vi "CAN_LIN_FlexRay_Demo_Template.vi"() -> ()   [LabVIEW 2014]
uses:
  TSMaster_API/LIN_Function/Typedef/TSLIN_Transmit.ctl
  TSMaster_API/CAN_CANFD_Function/Typedef/TLibCANFD.ctl
  TSMaster_API/LIN_Function/Typedef/TLibLIN.ctl
  TSMaster_API/FlexRay_Function/Typedef/TLibFLexRay.ctl
panel:
  out "FR_Buffer":T1[](array[typedef])
  out "ACANMsgBuffer":T2(array[cluster])
  out "ALINBuffer":T3[](array[typedef])
  # "使用方法：\n1.创建TSMaster 工程，映射CAN/LIN/FlexRay通道2，并开启接收Trace\n2.此demo 映射通道1\n3.通道1与通道2进行短接\n4.运行此demo 发送Fdata ,并接收Fdata"
  # "usage method:\n1. Create TSMaster project, map CAN/LIN/FlexRay channel 2, and enable receiving Trace. \n2. This demo maps channel 1. \n3. Short circuit channel 1 to channel 2\n4. Run this demo sends and receives Fdata"
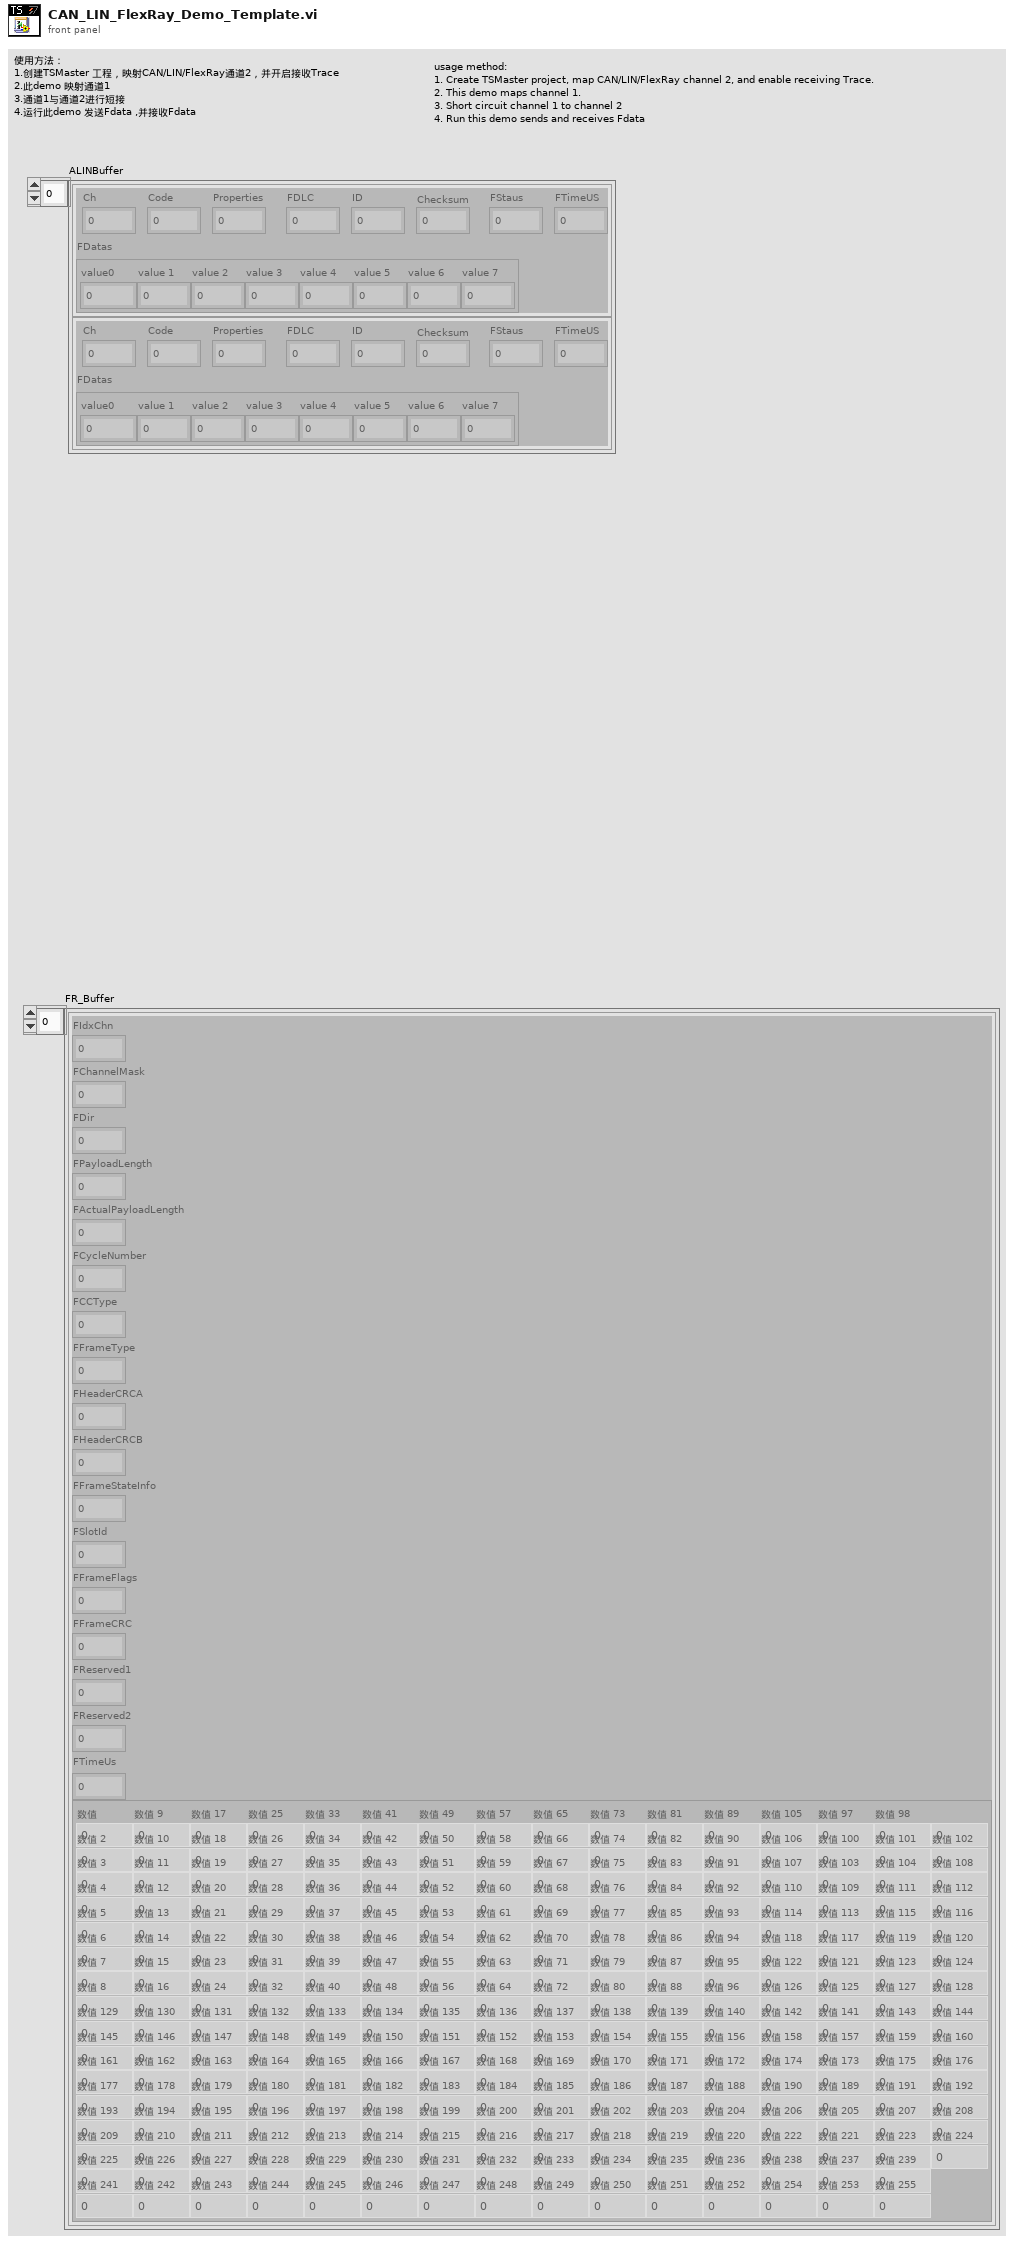
[diagram p1: front panel]
types:
  T1 = typedef "TLibFLexRay.ctl" = cluster{"FIdxChn":u8, "FChannelMask":u8, "FDir":u8, "FPayloadLength":u8, "FActualPayloadLength":u8, "FCycleNumber":u8, "FCCType":u8, "FFrameType":u8, "FHeaderCRCA":u16, "FHeaderCRCB":u16, "FFrameStateInfo":u16, "FSlotId":u16, "FFrameFlags":u32, "FFrameCRC":u32, "FReserved1":u64, "FReserved2":u64, "FTimeUs":u64, "FData":cluster{"数值":u8, "数值 9":u8, "数值 17":u8, "数值 25":u8, "数值 33":u8, "数值 41":u8, "数值 49":u8, "数值 57":u8, "数值 65":u8, "数值 73":u8, "数值 81":u8, "数值 89":u8, "数值 97":u8, "数值 105":u8, "数值 98":u8, "数值 99":u8, "数值 2":u8, "数值 10":u8, "数值 18":u8, "数值 26":u8, "数值 34":u8, "数值 42":u8, "数值 50":u8, "数值 58":u8, "数值 66":u8, "数值 74":u8, "数值 82":u8, "数值 90":u8, "数值 100":u8, "数值 106":u8, "数值 101":u8, "数值 102":u8, "数值 3":u8, "数值 11":u8, "数值 19":u8, "数值 27":u8, "数值 35":u8, "数值 43":u8, "数值 51":u8, "数值 59":u8, "数值 67":u8, "数值 75":u8, "数值 83":u8, "数值 91":u8, "数值 103":u8, "数值 107":u8, "数值 104":u8, "数值 108":u8, "数值 4":u8, "数值 12":u8, "数值 20":u8, "数值 28":u8, "数值 36":u8, "数值 44":u8, "数值 52":u8, "数值 60":u8, "数值 68":u8, "数值 76":u8, "数值 84":u8, "数值 92":u8, "数值 109":u8, "数值 110":u8, "数值 111":u8, "数值 112":u8, "数值 5":u8, "数值 13":u8, "数值 21":u8, "数值 29":u8, "数值 37":u8, "数值 45":u8, "数值 53":u8, "数值 61":u8, "数值 69":u8, "数值 77":u8, "数值 85":u8, "数值 93":u8, "数值 113":u8, "数值 114":u8, "数值 115":u8, "数值 116":u8, "数值 6":u8, "数值 14":u8, "数值 22":u8, "数值 30":u8, "数值 38":u8, "数值 46":u8, "数值 54":u8, "数值 62":u8, "数值 70":u8, "数值 78":u8, "数值 86":u8, "数值 94":u8, "数值 117":u8, "数值 118":u8, "数值 119":u8, "数值 120":u8, "数值 7":u8, "数值 15":u8, "数值 23":u8, "数值 31":u8, "数值 39":u8, "数值 47":u8, "数值 55":u8, "数值 63":u8, "数值 71":u8, "数值 79":u8, "数值 87":u8, "数值 95":u8, "数值 121":u8, "数值 122":u8, "数值 123":u8, "数值 124":u8, "数值 8":u8, "数值 16":u8, "数值 24":u8, "数值 32":u8, "数值 40":u8, "数值 48":u8, "数值 56":u8, "数值 64":u8, "数值 72":u8, "数值 80":u8, "数值 88":u8, "数值 96":u8, "数值 125":u8, "数值 126":u8, "数值 127":u8, "数值 128":u8, "数值 129":u8, "数值 130":u8, "数值 131":u8, "数值 132":u8, "数值 133":u8, "数值 134":u8, "数值 135":u8, "数值 136":u8, "数值 137":u8, "数值 138":u8, "数值 139":u8, "数值 140":u8, "数值 141":u8, "数值 142":u8, "数值 143":u8, "数值 144":u8, "数值 145":u8, "数值 146":u8, "数值 147":u8, "数值 148":u8, "数值 149":u8, "数值 150":u8, "数值 151":u8, "数值 152":u8, "数值 153":u8, "数值 154":u8, "数值 155":u8, "数值 156":u8, "数值 157":u8, "数值 158":u8, "数值 159":u8, "数值 160":u8, "数值 161":u8, "数值 162":u8, "数值 163":u8, "数值 164":u8, "数值 165":u8, "数值 166":u8, "数值 167":u8, "数值 168":u8, "数值 169":u8, "数值 170":u8, "数值 171":u8, "数值 172":u8, "数值 173":u8, "数值 174":u8, "数值 175":u8, "数值 176":u8, "数值 177":u8, "数值 178":u8, "数值 179":u8, "数值 180":u8, "数值 181":u8, "数值 182":u8, "数值 183":u8, "数值 184":u8, "数值 185":u8, "数值 186":u8, "数值 187":u8, "数值 188":u8, "数值 189":u8, "数值 190":u8, "数值 191":u8, "数值 192":u8, "数值 193":u8, "数值 194":u8, "数值 195":u8, "数值 196":u8, "数值 197":u8, "数值 198":u8, "数值 199":u8, "数值 200":u8, "数值 201":u8, "数值 202":u8, "数值 203":u8, "数值 204":u8, "数值 205":u8, "数值 206":u8, "数值 207":u8, "数值 208":u8, "数值 209":u8, "数值 210":u8, "数值 211":u8, "数值 212":u8, "数值 213":u8, "数值 214":u8, "数值 215":u8, "数值 216":u8, "数值 217":u8, "数值 218":u8, "数值 219":u8, "数值 220":u8, "数值 221":u8, "数值 222":u8, "数值 223":u8, "数值 224":u8, "数值 225":u8, "数值 226":u8, "数值 227":u8, "数值 228":u8, "数值 229":u8, "数值 230":u8, "数值 231":u8, "数值 232":u8, "数值 233":u8, "数值 234":u8, "数值 235":u8, "数值 236":u8, "数值 237":u8, "数值 238":u8, "数值 239":u8, "数值 241":u8, "数值 242":u8, "数值 243":u8, "数值 244":u8, "数值 245":u8, "数值 246":u8, "数值 247":u8, "数值 248":u8, "数值 249":u8, "数值 250":u8, "数值 251":u8, "数值 252":u8, "数值 253":u8, "数值 254":u8, "数值 255":u8}}
  T2 = cluster{"FIdxChn":u8, "FProperties":u8, "FDLC":u8, "FReserved":u8, "FIdentifier":i32, "FTimeUS":u64, "Fdata":cluster{"初始化的数组[0]":u8, "初始化的数组[1]":u8, "初始化的数组[2]":u8, "初始化的数组[3]":u8, "初始化的数组[4]":u8, "初始化的数组[5]":u8, "初始化的数组[6]":u8, "初始化的数组[7]":u8, "初始化的数组[8]":u8, "初始化的数组[9]":u8, "初始化的数组[10]":u8, "初始化的数组[11]":u8, "初始化的数组[12]":u8, "初始化的数组[13]":u8, "初始化的数组[14]":u8, "初始化的数组[15]":u8, "初始化的数组[16]":u8, "初始化的数组[17]":u8, "初始化的数组[18]":u8, "初始化的数组[19]":u8, "初始化的数组[20]":u8, "初始化的数组[21]":u8, "初始化的数组[22]":u8, "初始化的数组[23]":u8, "初始化的数组[24]":u8, "初始化的数组[25]":u8, "初始化的数组[26]":u8, "初始化的数组[27]":u8, "初始化的数组[28]":u8, "初始化的数组[29]":u8, "初始化的数组[30]":u8, "初始化的数组[31]":u8, "初始化的数组[32]":u8, "初始化的数组[33]":u8, "初始化的数组[34]":u8, "初始化的数组[35]":u8, "初始化的数组[36]":u8, "初始化的数组[37]":u8, "初始化的数组[38]":u8, "初始化的数组[39]":u8, "初始化的数组[40]":u8, "初始化的数组[41]":u8, "初始化的数组[42]":u8, "初始化的数组[43]":u8, "初始化的数组[44]":u8, "初始化的数组[45]":u8, "初始化的数组[46]":u8, "初始化的数组[47]":u8, "初始化的数组[48]":u8, "初始化的数组[49]":u8, "初始化的数组[50]":u8, "初始化的数组[51]":u8, "初始化的数组[52]":u8, "初始化的数组[53]":u8, "初始化的数组[54]":u8, "初始化的数组[55]":u8, "初始化的数组[56]":u8, "初始化的数组[57]":u8, "初始化的数组[58]":u8, "初始化的数组[59]":u8, "初始化的数组[60]":u8, "初始化的数组[61]":u8, "初始化的数组[62]":u8, "初始化的数组[63]":u8}}[]
  T3 = typedef "TLibLIN.ctl" = cluster{"Ch":u8, "Code":u8, "Properties":u8, "FDLC":u8, "ID":u8, "Checksum":u8, "FStaus":u8, "FTimeUS":u64, "FDatas":cluster{"value0":u8, "value 1":u8, "value 2":u8, "value 3":u8, "value 4":u8, "value 5":u8, "value 6":u8, "value 7":u8}}
  T4 = cluster{"FIdxChn":u8, "FChannelMask":u8, "FActualPayloadLength":u8, "FCycleNumber":u8, "FSlotId":u16, "Send_Array":u8[]}
  T5 = enum16{"Only read received messages", "Receive&send messages"}
  T6 = typedef "TLibCANFD.ctl" = cluster{"AIdxchn":u8, "AId":i32, "AIsStd":u8, "BRS":enum16{"Close", "Open"}, "AIsData":u8, "ADLC":i32, "AIsFD":enum16{"Classic CAN Message", "FD CAN Message"}, "FDatas":cluster{"Initialize array[0]":u8, "Initialize array[1]":u8, "Initialize array[2]":u8, "Initialize array[3]":u8, "Initialize array[4]":u8, "Initialize array[5]":u8, "Initialize array[6]":u8, "Initialize array[7]":u8, "Initialize array[8]":u8, "Initialize array[9]":u8, "Initialize array[10]":u8, "Initialize array[11]":u8, "Initialize array[12]":u8, "Initialize array[13]":u8, "Initialize array[14]":u8, "Initialize array[15]":u8, "Initialize array[16]":u8, "Initialize array[17]":u8, "Initialize array[18]":u8, "Initialize array[19]":u8, "Initialize array[20]":u8, "Initialize array[21]":u8, "Initialize array[22]":u8, "Initialize array[23]":u8, "Initialize array[24]":u8, "Initialize array[25]":u8, "Initialize array[26]":u8, "Initialize array[27]":u8, "Initialize array[28]":u8, "Initialize array[29]":u8, "Initialize array[30]":u8, "Initialize array[31]":u8, "Initialize array[32]":u8, "Initialize array[33]":u8, "Initialize array[34]":u8, "Initialize array[35]":u8, "Initialize array[36]":u8, "Initialize array[37]":u8, "Initialize array[38]":u8, "Initialize array[39]":u8, "Initialize array[40]":u8, "Initialize array[41]":u8, "Initialize array[42]":u8, "Initialize array[43]":u8, "Initialize array[44]":u8, "Initialize array[45]":u8, "Initialize array[46]":u8, "Initialize array[47]":u8, "Initialize array[48]":u8, "Initialize array[49]":u8, "Initialize array[50]":u8, "Initialize array[51]":u8, "Initialize array[52]":u8, "Initialize array[53]":u8, "Initialize array[54]":u8, "Initialize array[55]":u8, "Initialize array[56]":u8, "Initialize array[57]":u8, "Initialize array[58]":u8, "Initialize array[59]":u8, "Initialize array[60]":u8, "Initialize array[61]":u8, "Initialize array[62]":u8, "Initialize array[63]":u8}}
  T7 = typedef "TSLIN_Transmit.ctl" = cluster{"Channel":i32, "Rx/TX":enum16{"Rx", "Tx"}, "Set_node_funtiontype":i32, "DLC":u32, "ID":u32, "FDatas":cluster{"value0":u8, "value 1":u8, "value 2":u8, "value 3":u8, "value 4":u8, "value 5":u8, "value 6":u8, "value 7":u8}}
  T8 = cluster{"数组[0]":u8, "数组[1]":u8, "数组[2]":u8, "数组[3]":u8, "数组[4]":u8, "数组[5]":u8, "数组[6]":u8, "数组[7]":u8, "数组[8]":u8, "数组[9]":u8, "数组[10]":u8, "数组[11]":u8, "数组[12]":u8, "数组[13]":u8, "数组[14]":u8, "数组[15]":u8, "数组[16]":u8, "数组[17]":u8, "数组[18]":u8, "数组[19]":u8, "数组[20]":u8, "数组[21]":u8, "数组[22]":u8, "数组[23]":u8, "数组[24]":u8, "数组[25]":u8, "数组[26]":u8, "数组[27]":u8, "数组[28]":u8, "数组[29]":u8, "数组[30]":u8, "数组[31]":u8, "数组[32]":u8, "数组[33]":u8, "数组[34]":u8, "数组[35]":u8, "数组[36]":u8, "数组[37]":u8, "数组[38]":u8, "数组[39]":u8, "数组[40]":u8, "数组[41]":u8, "数组[42]":u8, "数组[43]":u8, "数组[44]":u8, "数组[45]":u8, "数组[46]":u8, "数组[47]":u8, "数组[48]":u8, "数组[49]":u8, "数组[50]":u8, "数组[51]":u8, "数组[52]":u8, "数组[53]":u8, "数组[54]":u8, "数组[55]":u8, "数组[56]":u8, "数组[57]":u8, "数组[58]":u8, "数组[59]":u8, "数组[60]":u8, "数组[61]":u8, "数组[62]":u8, "数组[63]":u8}
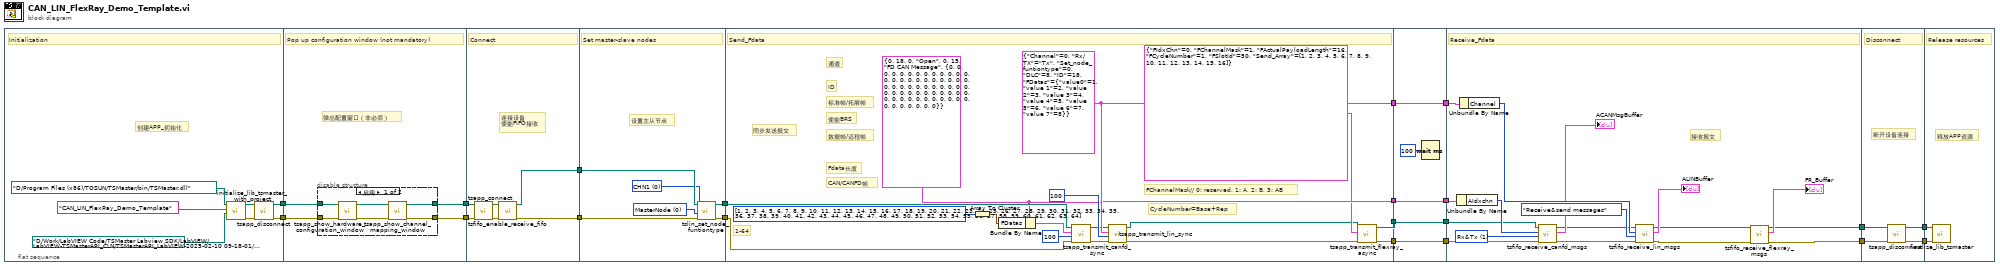
[diagram p0: block diagram]
diagram:
  n1 = flat-sequence {
    tunnel: [w27] -> w20
    tunnel: [w26] -> w19
    tunnel: w20 -> [w31]
    tunnel: w19 -> [w30]
    tunnel: [w29] -> w10
    tunnel: [w28] -> w9
    tunnel: [w43] -> w18
    tunnel: [w42] -> w17
    tunnel: w10 -> [w41]
    tunnel: w9 -> [w40]
    tunnel: w18 -> [w51]
    tunnel: w17 -> [w50]
    tunnel: [w48] -> w16
    tunnel: [w47] -> w15
    tunnel: w16 -> [w61]
    tunnel: w15 -> [w60]
    tunnel: [w54] -> w8
    tunnel: [w52] -> w6
    tunnel: [w66] -> w4
    tunnel: [w57] -> w2
    tunnel: w8 -> [w72]
    tunnel: [w72] -> w7
    tunnel: w6 -> [w71]
    tunnel: [w71] -> w5
    tunnel: w4 -> [w70]
    tunnel: [w70] -> w3
    tunnel: w2 -> [w69]
    tunnel: [w69] -> w1
    tunnel: w7 -> [w81]
    tunnel: w5 -> [w80]
    tunnel: w3 -> [w89]
    tunnel: [w74] -> w14
    tunnel: [w73] -> w13
    tunnel: w1 -> [w82]
    tunnel: w14 -> [w93]
    tunnel: w13 -> [w92]
    tunnel: [w91] -> w12
    tunnel: [w90] -> w11
    tunnel: w12 -> [w95]
    tunnel: w11 -> [w94]
    frame #0 {
      # "创建APP_初始化"
      # "Initialization"
      n2 = call "initialize_lib_tsmaster_with_project.vi"("projectfile"=path "D:/Work/LabVIEW Code/TSMaster Labview SDK/LabVIEW/LabVIEW-TSMasterAPI_CLN/TSMasterAPI_LabVIEW-2025-02-10 09-18-01/Demo/CAN_LIN_FlexRay/TSMaster_CAN_LIN_FlexRay", "AppName"="CAN_LIN_FlexRay_Demo_Template", "Path input"=path "D:/Program Files (x86)/TOSUN/TSMaster/bin/TSMaster.dll") -> ("error output"=w21:errorcluster, "Path output"=w22:path)  [unwired: 7 in]
      n3 = call "tsapp_disconnect.vi"("error in (no error)"=w21, "Path"=w22) -> ("error output"=w26:errorcluster, "Path output"=w27:path)  [unwired: 7 in, 1 out]
    }
    frame #1 {
      # "弹出配置窗口（非必须）"
      # "Pop up configuration window (not mandatory)"
      n4 = disable-structure shown="启用" {
        disable-tunnel: w31 -> [w37 w39]
        disable-tunnel: w30 -> [w36 w38]
        disable-tunnel: [w33 w39] -> w29
        disable-tunnel: [w32 w38] -> w28
        frame Enabled {
          n5 = call "tsapp_show_hardware_configuration_window.vi"("error in (no error)"=w36, "路径输入"=w37) -> ("error out"=w34:errorcluster, "路径输出"=w35:path)  [unwired: 7 in, 1 out]
          n6 = call "tsapp_show_channel_mapping_window.vi"("error in (no error)"=w34, "路径输入"=w35) -> ("error out"=w32:errorcluster, "路径输出"=w33:path)  [unwired: 7 in, 1 out]
        }
        frame Disabled {
        }
      }
    }
    frame #2 {
      # "连接设备\n使能FIFO接收"
      # "Connect"
      n7 = call "tsapp_connect.vi"("error in (no error)"=w40, "Path"=w41) -> ("error out"=w45:errorcluster, "Path output"=w44:path)  [unwired: 7 in, 1 out]
      n8 = call "tsfifo_enable_receive_fifo.vi"("error in (no error)"=w45, "Path"=w44) -> ("error out"=w42:errorcluster, "Path output"=w43:path)  [unwired: 8 in]
    }
    frame #3 {
      w46 = 0 items=["CHN1", "CHN2", "CHN3", "CHN4", "CHN5", "CHN6", "CHN7", "CHN8", "CHN9", "CHN10", "CHN11", "CHN12", "CHN13", "CHN14", "CHN15", "CHN16", "CHN17", "CHN18", "CHN19", "CHN20", "CHN21", "CHN22", "CHN23", "CHN24", "CHN25", "CHN26", "CHN27", "CHN28", "CHN29", "CHN30", "CHN31", "CHN32"] ("AAppChannel")
      w49 = 0 items=["MasterNode", "SlaveNode", "MonitorNote"] ("set_node_funtiontype")
      # "设置主从节点"
      # "Set master-slave nodes"
      n9 = call "tslin_set_node_funtiontype.vi"("错误输入（无错误）"=w50, "set_node_funtiontype"=w49, "AAppChannel"=w46, "path"=w51) -> ("错误输出"=w47:errorcluster, "path out"=w48:path)  [unwired: 5 in, 1 out]
    }
    frame #4 {
      w57 = T6 {"AIdxchn"=0, "AId"=18, "AIsStd"=0, "BRS"=enum."Open", "AIsData"=0, "ADLC"=15, "AIsFD"=enum."FD CAN Message", "FDatas"={"Initialize array[0]"=0, "Initialize array[1]"=0, "Initialize array[2]"=0, "Initialize array[3]"=0, "Initialize array[4]"=0, "Initialize array[5]"=0, "Initialize array[6]"=0, "Initialize array[7]"=0, "Initialize array[8]"=0, "Initialize array[9]"=0, "Initialize array[10]"=0, "Initialize array[11]"=0, "Initialize array[12]"=0, "Initialize array[13]"=0, "Initialize array[14]"=0, "Initialize array[15]"=0, "Initialize array[16]"=0, "Initialize array[17]"=0, "Initialize array[18]"=0, "Initialize array[19]"=0, "Initialize array[20]"=0, "Initialize array[21]"=0, "Initialize array[22]"=0, "Initialize array[23]"=0, "Initialize array[24]"=0, "Initialize array[25]"=0, "Initialize array[26]"=0, "Initialize array[27]"=0, "Initialize array[28]"=0, "Initialize array[29]"=0, "Initialize array[30]"=0, "Initialize array[31]"=0, "Initialize array[32]"=0, "Initialize array[33]"=0, "Initialize array[34]"=0, "Initialize array[35]"=0, "Initialize array[36]"=0, "Initialize array[37]"=0, "Initialize array[38]"=0, "Initialize array[39]"=0, "Initialize array[40]"=0, "Initialize array[41]"=0, "Initialize array[42]"=0, "Initialize array[43]"=0, "Initialize array[44]"=0, "Initialize array[45]"=0, "Initialize array[46]"=0, "Initialize array[47]"=0, "Initialize array[48]"=0, "Initialize array[49]"=0, "Initialize array[50]"=0, "Initialize array[51]"=0, "Initialize array[52]"=0, "Initialize array[53]"=0, "Initialize array[54]"=0, "Initialize array[55]"=0, "Initialize array[56]"=0, "Initialize array[57]"=0, "Initialize array[58]"=0, "Initialize array[59]"=0, "Initialize array[60]"=0, "Initialize array[61]"=0, "Initialize array[62]"=0, "Initialize array[63]"=0}} ("TCANFD")
      w66 = T7 {"Channel"=0, "Rx/TX"=enum."Tx", "Set_node_funtiontype"=0, "DLC"=8, "ID"=18, "FDatas"={"value0"=1, "value 1"=2, "value 2"=3, "value 3"=4, "value 4"=5, "value 5"=6, "value 6"=7, "value 7"=8}} ("LIN_Transmit")
      # "CycleNumber=Base+Rep"
      # "FChannelMask// 0: reserved, 1: A, 2: B, 3: AB"
      # "CAN/CANFD帧"
      # "Fdata长度"
      # "数据帧/远程帧"
      # "使能BRS"
      # "标准帧/拓展帧"
      # "ID"
      # "通道"
      # "1-64"
      # "同步发送报文"
      # "Send_Fdata"
      n10 = Array To Cluster(array=u8[] [1, 2, 3, 4, 5, 6, 7, 8, 9, 10, 11, 12, 13, 14, 15, 16, 17, 18, 19, 20, 21, 22, 23, 24, 25, 26, 27, 28, 29, 30, 31, 32, 33, 34, 35, 36, 37, 38, 39, 40, 41, 42, 43, 44, 45, 46, 47, 48, 49, 50, 51, 52, 53, 54, 55, 56, 57, 58, 59, 60, 61, 62, 63, 64] ("数组")) -> (cluster=w64:T8)
      n11 = Bundle By Name(cluster=w57, "FDatas"=w64) -> (w63:T6)
      n12 = call "tsapp_transmit_canfd_sync.vi"("error in (no error)"=w60, "ATimeoutMS"=100, "TCANFD"=w63, "Path"=w61) -> ("error out"=w58:errorcluster, "Path output"=w59:path)  [unwired: 5 in, 1 out]
      n13 = call "tsapp_transmit_lin_sync.vi"("错误输入（无错误）"=w58, "ATimeoutMS"=100, "LIN_Transmit"=w66, "路径输入"=w59) -> ("错误输出"=w53:errorcluster, "路径输出"=w55:path)  [unwired: 5 in, 1 out]
      n14 = call "tsapp_transmit_flexray_async.vi"("error in (no error)"=w53, "FR_Transmit"=T4 {"FIdxChn"=0, "FChannelMask"=1, "FActualPayloadLength"=16, "FCycleNumber"=1, "FSlotId"=50, "Send_Array"=[1, 2, 3, 4, 5, 6, 7, 8, 9, 10, 11, 12, 13, 14, 15, 16]}, "Path"=w55) -> ("error out"=w52:errorcluster, "Path output"=w54:path)  [unwired: 5 in, 1 out]
    }
    frame #5 {
      n15 = Wait (ms)(milliseconds to wait=u32 100 ("等待时间（毫秒）")) -> ()  [unwired: 1 out]
    }
    frame #6 {
      w84 = u16 1 items=["Rx", "Rx&Tx"] ("Display message type")
      # "接收报文"
      # "Receive_Fdata"
      n16 = Unbundle By Name(w82) -> ("AIdxchn"=w85:u8)
      n17 = Unbundle By Name(w89) -> ("Channel"=w88:i32)
      n18 = call "tsfifo_receive_canfd_msgs.vi"("error in (no error)"=w80, "Display message type"=w84, "AAPPChannel"=w85, "Path"=w81) -> ("error out"=w78:errorcluster, "ACANMsgBuffer"=→"ACANMsgBuffer":T2, "Path output"=w79:path)  [unwired: 3 in, 1 out]
      n19 = call "tsfifo_receive_lin_msgs.vi"("错误输入（无错误）"=w78, "Read message type"=T5."Receive&send messages", "AIdxChn"=w88, "路径输入"=w79) -> ("错误输出"=w75:errorcluster, "ALINBuffer"=→"ALINBuffer":T3[], "路径输出"=w76:path)  [unwired: 4 in, 1 out]
      n20 = call "tsfifo_receive_flexray_msgs.vi"("error in (no error)"=w75, "Path"=w76) -> ("error out"=w73:errorcluster, "FR_Buffer"=→"FR_Buffer":T1[], "Path output"=w74:path)  [unwired: 5 in, 1 out]
    }
    frame #7 {
      # "断开设备连接"
      # "Disconnect"
      n21 = call "tsapp_disconnect.vi"("error in (no error)"=w92, "Path"=w93) -> ("error output"=w91:errorcluster, "Path output"=w90:path)  [unwired: 7 in, 1 out]
    }
    frame #8 {
      # "释放APP资源"
      # "Release resources"
      n22 = call "finalize_lib_tsmaster.vi"("error in (no error)"=w95, "Path"=w94) -> ()  [unwired: 8 in, 2 out]
    }
  }
